vi "ConnectionHelperVMXTitan.vi"(5 "InCluster":cluster{"Motors":dbl[], "HCDIOValues":dbl[]}, 6 "ErrorIn":errorcluster, 9 "Reference":T1) -> (0 "ErrorOut":errorcluster, 3 "OutReference":T1, 4 "OutCluster":T3)   [LabVIEW 2019]
uses:
  <vilib>/vision/Image Controls.llb/IMAQ Image.ctl
  C:/Users/user/Desktop/lvlib/assemblies/x86/LibraryForLabVIEW.dll
  assemblies/x86/LibraryForLabVIEW.dll
  <vilib>/Utility/importsl/GetValueByPointer/datatype.ctl
  <vilib>/Utility/importsl/GetValueByPointer/GetValueByPointer.xnode
panel:
  out "size(s) 2":i32
  out "size(s)":i32
  out "Array":u8[](array[numeric])
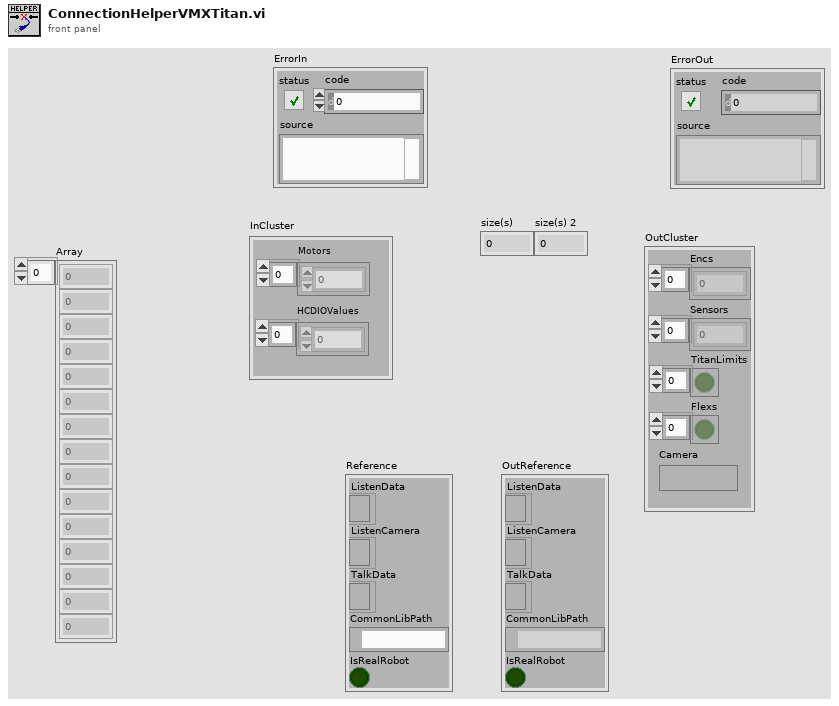
[diagram p1: front panel]
types:
  T1 = cluster{"ListenData":refnum<k24>, "ListenCamera":refnum<k24>, "TalkData":refnum<k24>, "CommonLibPath":path, "IsRealRobot":bool}
  T2 = typedef "IMAQ Image.ctl" = refnum<image>
  T3 = cluster{"Encs":dbl[], "Sensors":dbl[], "TitanLimits":bool[], "Flexs":bool[], "Camera":T2}
  T4 = enum32{"pack1", "pack2", "pack4", "pack8", "pack16"}
  T5 = typedef "Image Type" = u32
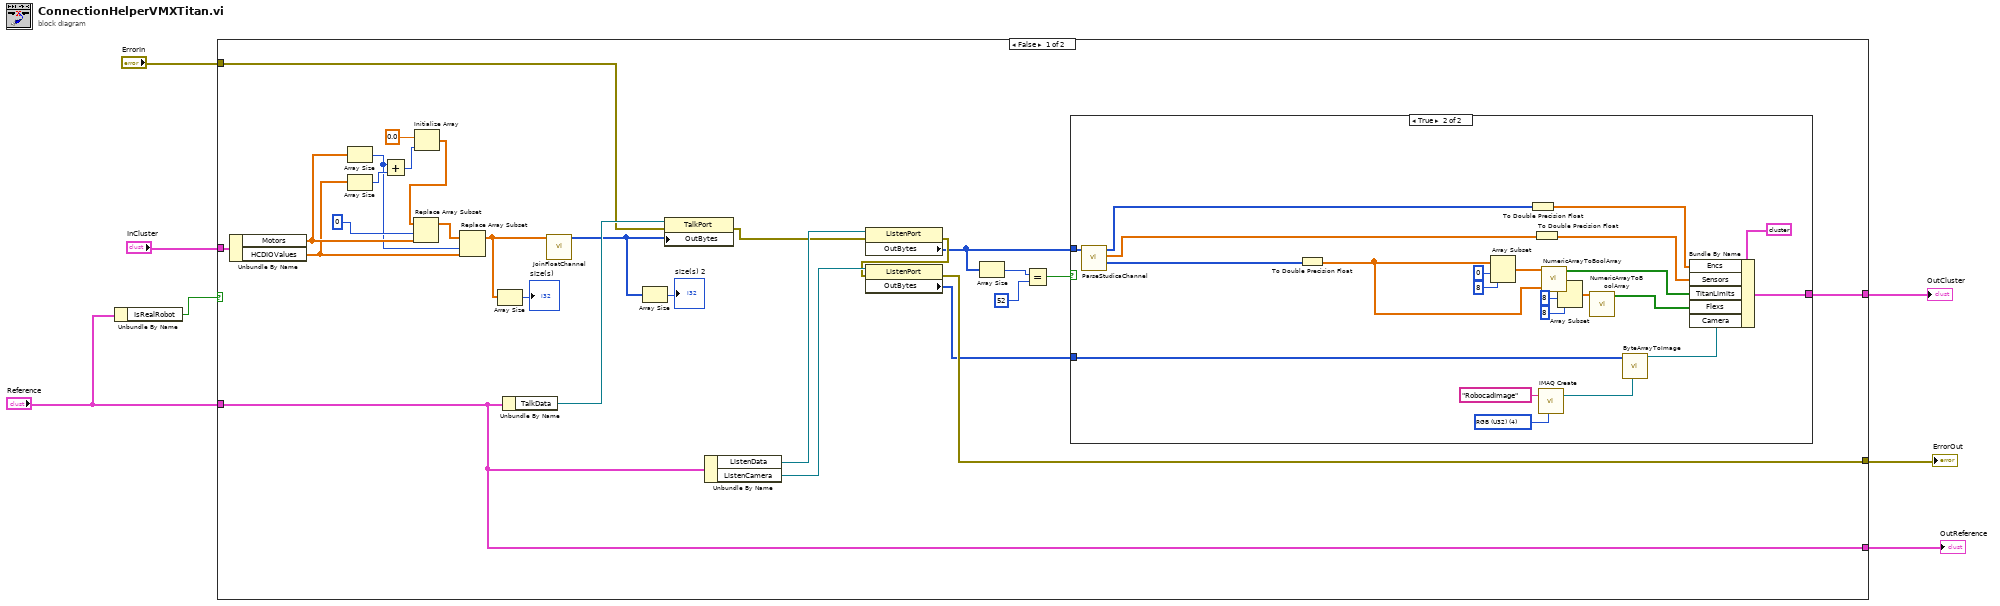
[diagram p0: block diagram]
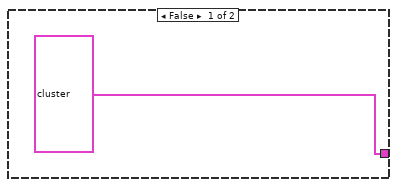
[diagram p2: hidden frame]
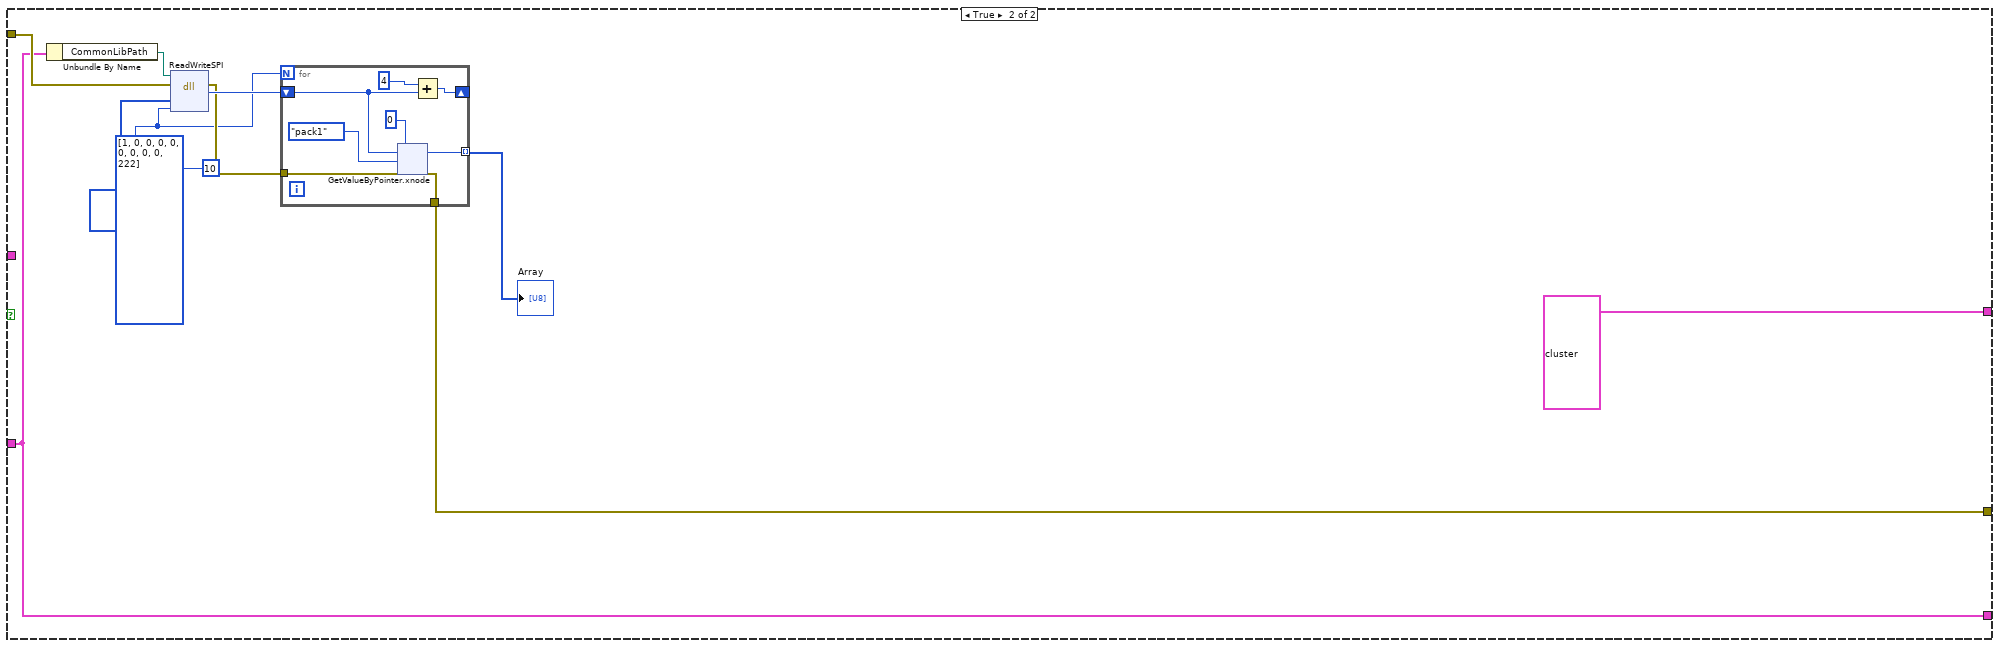
[diagram p3: hidden frame]
diagram:
  n1 = Unbundle By Name("Reference") -> ("IsRealRobot"=w1:bool)
  n2 = case shown="False" w1 {
    tunnel: "InCluster" -> [w35 _]
    tunnel: "ErrorIn" -> [w33 w65]
    tunnel: [w31 w61] -> w5
    tunnel: [w18 T3 {"Encs"=[], "Sensors"=[], "TitanLimits"=[], "Flexs"=[], "Camera"=refnum} ("OutCluster")] -> w4
    tunnel: "Reference" -> [w16 w59]
    tunnel: [w16 w59] -> w3
    frame False {
      n3 = Unbundle By Name(w35) -> ("Motors"=w23:dbl[], "HCDIOValues"=w20:dbl[])
      n4 = Array Size(array=w23) -> (size(s)=w19:i32)
      n5 = Array Size(array=w20) -> (size(s)=w26:i32)
      n6 = Add(x=w19, y=w26) -> (x+y=w25:i32)
      n7 = Initialize Array(0.0 ("element"), w25) -> (w24:dbl[])
      n8 = Replace Array Subset(array=w24, new element=w23, index=0) -> (w21:dbl[])
      n9 = Replace Array Subset(array=w21, new element=w20, index=w19) -> (w11:dbl[])
      n10 = Array Size(array=w11) -> (size(s)=→"size(s)":i32)
      n11 = Unbundle By Name(w16) -> ("TalkData"=w34:refnum<k24>)
      n12 = call "JoinFloatChannel.vi"("Array"=w11) -> ("OutArray"=w9:u8[])  [unwired: 10 in]
      n13 = Array Size(array=w9) -> (size(s)=→"size(s) 2":i32)
      n14 = property class="TalkPort"(reference=w34, error in=w33, "OutBytes"=w9) -> (error out=w28:errorcluster)  [unwired: 1 out]
      n15 = Unbundle By Name(w16) -> ("ListenData"=w32:refnum<k24>, "ListenCamera"=w30:refnum<k24>)
      n16 = property class="ListenPort"(reference=w32, error in=w28) -> (error out=w29:errorcluster, "OutBytes"=w15:u8[])  [unwired: 1 out]
      n17 = property class="ListenPort"(reference=w30, error in=w29) -> (error out=w31:errorcluster, "OutBytes"=w17:u8[])  [unwired: 1 out]
      n18 = Array Size(array=w15) -> (size(s)=w13:i32)
      n19 = Equal?(x=w13, y=52) -> (x = y?=w14:bool)
      n20 = case shown="True" w14 {
        tunnel: [T3 {"Encs"=[], "Sensors"=[], "TitanLimits"=[], "Flexs"=[], "Camera"=refnum} ("OutCluster") w57] -> w18
        tunnel: w17 -> [_ w55]
        tunnel: w15 -> [_ w43]
        frame False {
        }
        frame True {
          w54 = T5 4 items=["Grayscale (U8)", "Grayscale (I16)", "Grayscale (SGL)", "Complex (CSG)", "RGB (U32)", "HSL (U32)", "RGB (U64)", "Grayscale (U16)"] ("Image Type")
          n21 = call "ParseStudicaChannel.vi"("Array"=w43) -> ("ButtonsAndOther"=w37:u8[], "Sensors"=w40:sgl[], "Encs"=w42:i32[])  [unwired: 8 in]
          n22 = To Double Precision Float(number=w37) -> (double precision float=w38:dbl[])
          n23 = Array Subset(array=w38, index=0, length=8) -> (w49:dbl[])
          n24 = To Double Precision Float(number=w42) -> (double precision float=w41:dbl[])
          n25 = To Double Precision Float(number=w40) -> (double precision float=w39:dbl[])
          n26 = call "IMAQ Create"("Image Name"="RobocadImage", "Image Type"=w54) -> ("New Image"=w52:T2)  [unwired: 3 in, 1 out]
          n27 = call "NumericArrayToBoolArray.vi"("InArray"=w49) -> ("OutArray"=w48:bool[])  [unwired: 10 in]
          n28 = Array Subset(array=w38, index=8, length=8) -> (w45:dbl[])
          n29 = call "NumericArrayToBoolArray.vi"("InArray"=w45) -> ("OutArray"=w44:bool[])  [unwired: 10 in]
          n30 = call "ByteArrayToImage.vi"("CameraBytes"=w55, "Image"=w52) -> ("Image Out"=w56:T2)  [unwired: 6 in]
          n31 = Bundle By Name(cluster=T3 {"Encs"=[], "Sensors"=[], "TitanLimits"=[], "Flexs"=[], "Camera"=refnum} ("OutCluster"), "Encs"=w41, "Sensors"=w39, "TitanLimits"=w48, "Flexs"=w44, "Camera"=w56) -> (w57:T3)
        }
      }
    }
    frame True {
      w62 = u8 10
      n32 = Unbundle By Name(w59) -> ("CommonLibPath"=w66:path)
      n33 = dll-call lib="?" fn="ReadWriteSPI"(path in=w66, error in=w65, "data"=u8[] [1, 0, 0, 0, 0, 0, 0, 0, 0, 222], "len"=w62) -> (error out=w64:errorcluster, "return type"=w68:u64)  [unwired: 3 in, 1 out]
      n34 = for {
        N: w62 -> [_]
        tunnel: [w74] -> w67 mode=indexing
        shift-right: [w73] -> _
        shift-left: w68 -> [w72]
        tunnel: w64 -> [w70]
        tunnel: [w69] -> w61
        n35 = xnode "GetValueByPointer.xnode"("Pointer"=w72, "InputType"=u8 0, "PackType"=T4."pack1", "ErrorIn"=w70) -> ("Output"=w74:u8, "ErrorOut"=w69:errorcluster)
        n36 = Add(x=u64 4, y=w72) -> (x+y=w73:u64)
      }
      "Array" <- w67
    }
  }
  "ErrorOut" <- w5
  "OutCluster" <- w4
  "OutReference" <- w3
